vi "整合数据10.vi"(7 "Data in":i32[](array[numeric])) -> (1 "P1":i16, 2 "I1":i16, 3 "D1":i16, 4 "P2":i16, 6 "I2":i16, 10 "D2":i16, 12 "10":i16, 13 "D3":i16, 14 "I3":i16, 15 "P3":i16)   [LabVIEW 2016]
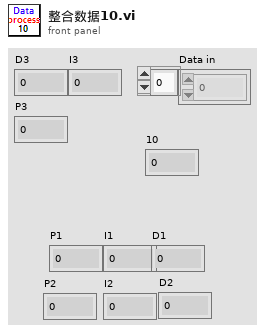
[diagram p1: front panel]
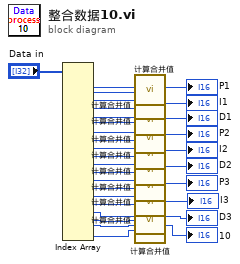
[diagram p0: block diagram]
diagram:
  n1 = Index Array(array="Data in") -> (element #1=w21:i32, element #2=w20:i32, element #3=w19:i32, element #4=w18:i32, element #5=w17:i32, element #6=w16:i32, element #7=w15:i32, element #8=w14:i32, element #9=w13:i32, element #10=w12:i32, element #11=w11:i32, element #12=w10:i32, element #13=w9:i32, element #14=w8:i32, element #15=w7:i32, element #16=w6:i32, element #17=w5:i32, element #18=w4:i32, element #19=w2:i32, element #20=w1:i32)  [unwired: 20 in]
  n2 = call "计算合并值.vi"("数值H"=w21, "数值L"=w20) -> ("合并数值"=→"P1":i16)  [unwired: 17 in]
  n3 = call "计算合并值.vi"("数值H"=w19, "数值L"=w18) -> ("合并数值"=→"I1":i16)  [unwired: 17 in]
  n4 = call "计算合并值.vi"("数值H"=w17, "数值L"=w16) -> ("合并数值"=→"D1":i16)  [unwired: 17 in]
  n5 = call "计算合并值.vi"("数值H"=w15, "数值L"=w14) -> ("合并数值"=→"P2":i16)  [unwired: 17 in]
  n6 = call "计算合并值.vi"("数值H"=w13, "数值L"=w12) -> ("合并数值"=→"I2":i16)  [unwired: 17 in]
  n7 = call "计算合并值.vi"("数值H"=w11, "数值L"=w10) -> ("合并数值"=→"D2":i16)  [unwired: 17 in]
  n8 = call "计算合并值.vi"("数值H"=w9, "数值L"=w8) -> ("合并数值"=→"P3":i16)  [unwired: 17 in]
  n9 = call "计算合并值.vi"("数值H"=w7, "数值L"=w6) -> ("合并数值"=→"I3":i16)  [unwired: 17 in]
  n10 = call "计算合并值.vi"("数值H"=w5, "数值L"=w4) -> ("合并数值"=→"D3":i16)  [unwired: 17 in]
  n11 = call "计算合并值.vi"("数值H"=w2, "数值L"=w1) -> ("合并数值"=→"10":i16)  [unwired: 17 in]
